vi "specu1a 1.0.0 Open Device Class.vi"(3 "error in":errorcluster, 5 "specu1a 1.0.0 Model Name":T1) -> (0 "error out":errorcluster, 2 "Device Handle":i32)   [LabVIEW 2010]
uses:
  Controls/specu1a 1.0.0 Model Class.ctl
  WINDOWS/SYSTEM32/DRIVERS/specu1a.dll
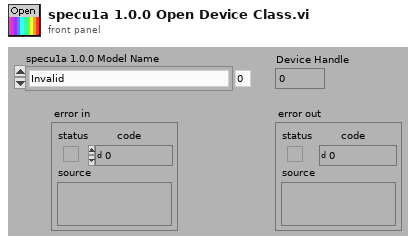
[diagram p1: front panel]
types:
  T1 = typedef "specu1a 1.0.0 Model Class.ctl" = enum16{"Invalid", "TG-NIR or SWNIR or UV", "TG-COOLED NIR-I or II", "TM-UV/VIS or VIS/NIR", "TM-UV/VIS or VIS/NIR CCD1 or CCD2", "RC- Vis or SWNIR Module"}
  T2 = typedef "specu1a 1.0.0 Error codes.ctl" = enum16{"INVALID_HANDLE_VALUE", "USBDEV_SUCCESS", "USBDEV_INVALID_HANDLE", "USBDEV_UNSUCCESS", "USBDEV_INVALID_VALUE", "USBDEV_CHECK_NORMAL", "USBDEV_CHECK_INVALID", "USBDEV_CHECK_REMOVE", "USBDEV_CHECK_OTHER", "USBDEV_RESET_ERROR", "USBDEV_BULKSIZE_ERROR", "USBDEV_BULK_READ_ERROR", "USBDEV_BULK_NOT_UPDATED", "USBDEV_TIME_OVER_ERROR", "USBDEV_TIME_UNDER_ERROR", "USBDEV_TIME_SET_ERROR", "USBDEV_SET_GAIN_ERROR", "USBDEV_GET_TEMP_ERROR", "USBDEV_SET_TRIGGER_ERROR", "USBDEV_RW_EEP_ADDR_ERROR", "USBDEV_RW_EEP_SIZE_ERROR", "USBDEV_RW_EEP_OVER_ERROR", "USBDEV_RW_EEP_ERROR", "UNITID_PRODUCTID_CONFLICT", "UNKNOWN_ERROR"}
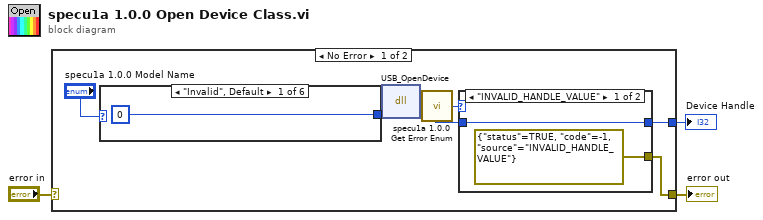
[diagram p0: block diagram]
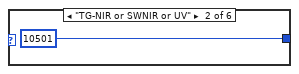
[diagram p2: hidden frame]
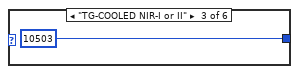
[diagram p3: hidden frame]
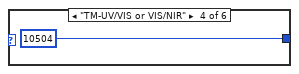
[diagram p4: hidden frame]
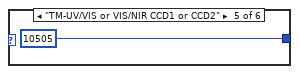
[diagram p5: hidden frame]
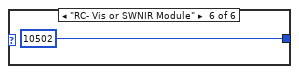
[diagram p6: hidden frame]
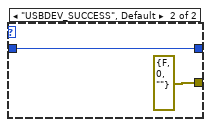
[diagram p7: hidden frame]
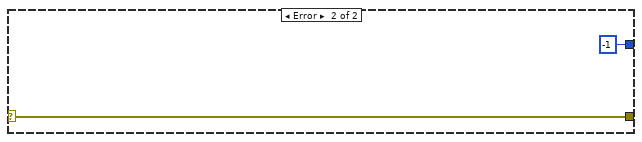
[diagram p8: hidden frame]
diagram:
  n1 = case shown="No Error" "error in" {
    selector: "error in" -> [_ w21]
    tunnel: [w9 w21] -> w3
    tunnel: [w8 -1 ("Device Handle")] -> w2
    frame No Error {
      n2 = case shown="\"Invalid\", Default" "specu1a 1.0.0 Model Name" {
        tunnel: [u16 0 u16 10501 u16 10503 u16 10504 u16 10505 u16 10502] -> w4
        frame "Invalid", Default {
        }
        frame "TG-NIR or SWNIR or UV" {
        }
        frame "TG-COOLED NIR-I or II" {
        }
        frame "TM-UV/VIS or VIS/NIR" {
        }
        frame "TM-UV/VIS or VIS/NIR CCD1 or CCD2" {
        }
        frame "RC- Vis or SWNIR Module" {
        }
      }
      n3 = dll-call lib="C:/WINDOWS/SYSTEM32/DRIVERS/specu1a.dll" fn="USB_OpenDevice" label="1.0.0 Open Device"("ProductID"=w4) -> (w6:i32)  [unwired: 4 in, 2 out]
      n4 = call "specu1a 1.0.0 Get Error Enum.vi"("Error Code in"=w6) -> ("Specu1a 1.0.0 Error code out"=w7:T2)  [unwired: 4 in]
      n5 = case shown="\"INVALID_HANDLE_VALUE\"" w7 {
        tunnel: [w16 w18] -> w8
        tunnel: [errorcluster {"status"=TRUE, "code"=-1, "source"="INVALID_HANDLE_VALUE"} ("error out") errorcluster {"status"=FALSE, "code"=0, "source"=""} ("error out")] -> w9
        tunnel: w6 -> [w16 w18]
        frame "INVALID_HANDLE_VALUE" {
        }
        frame "USBDEV_SUCCESS", Default {
        }
      }
    }
    frame Error {
    }
  }
  "error out" <- w3
  "Device Handle" <- w2
